vi "Auto_guider_queued.vi"() -> ()   [LabVIEW 2018]
uses:
  Global_Telescopio.vi
panel:
  out "respQ":refnum<queue>
  out "cmdQ":refnum<queue>
  in  "Case Constant\n(See Context Help) 2":bool
  in  "Case Constant\n(See Context Help)":bool=TRUE
  out "substring 3":string
  out "substring 2":string
  out "concatenated string":string
  out "substring":string
  out "result string":string
  in  "esc_placa":string="0.462"
  in  "guide_esp":string="S"
  in  "guide_cas":string="S"
  in  "guide_str":string="04/10/09  1:18:34\u000013 27 13\u0000-12 45 20\u0000"
  in  "guide_ang":string=" 281.52"
  in  "guide_nor":string="  11.53"
  in  "Tx_sts":u8[](array[numeric])=[22, 2, 1, 0, 83, 0, 0]
  out "rxsts 3":bool
  in  "SYN | ETX":u8[](array[numeric])=[22, 3] format="%02.0f"
  in  "tel_sts2":u8[](array[numeric])=[0, 0, 0] format="%02.0f"
  in  "Tx_ena":u8[](array[numeric])=[22, 2, 1, 0, 72, 0, 0] format="%02.0f"
  out "tel_sts1":bool[](array[boolean])=[TRUE, TRUE, TRUE, TRUE, FALSE, FALSE, TRUE]
  out "guide_dec":dbl format="%07.2g"
  out "guide_dir_ns":string
  out "guide_asc":dbl format="%07.2g"
  out "guide_dir_we":string
  in  "SYN | ACK":u8[](array[numeric])=[22, 6] format="%02.0f"
  out "rxsts":bool
  in  "Tx_nak":u8[](array[numeric])=[22, 21]
  out "Data rx guider":string
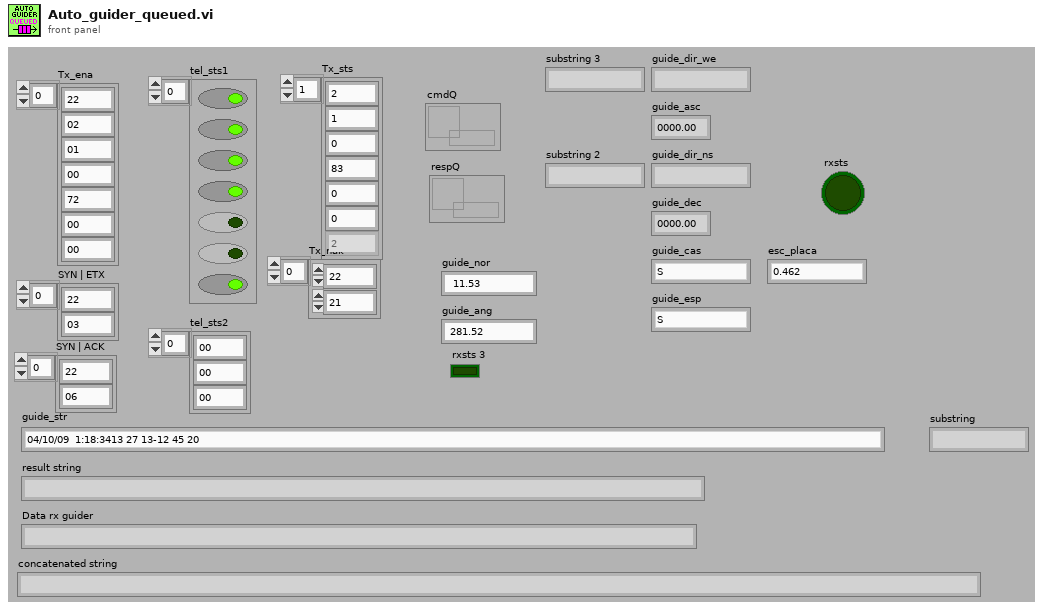
[diagram p1: front panel]
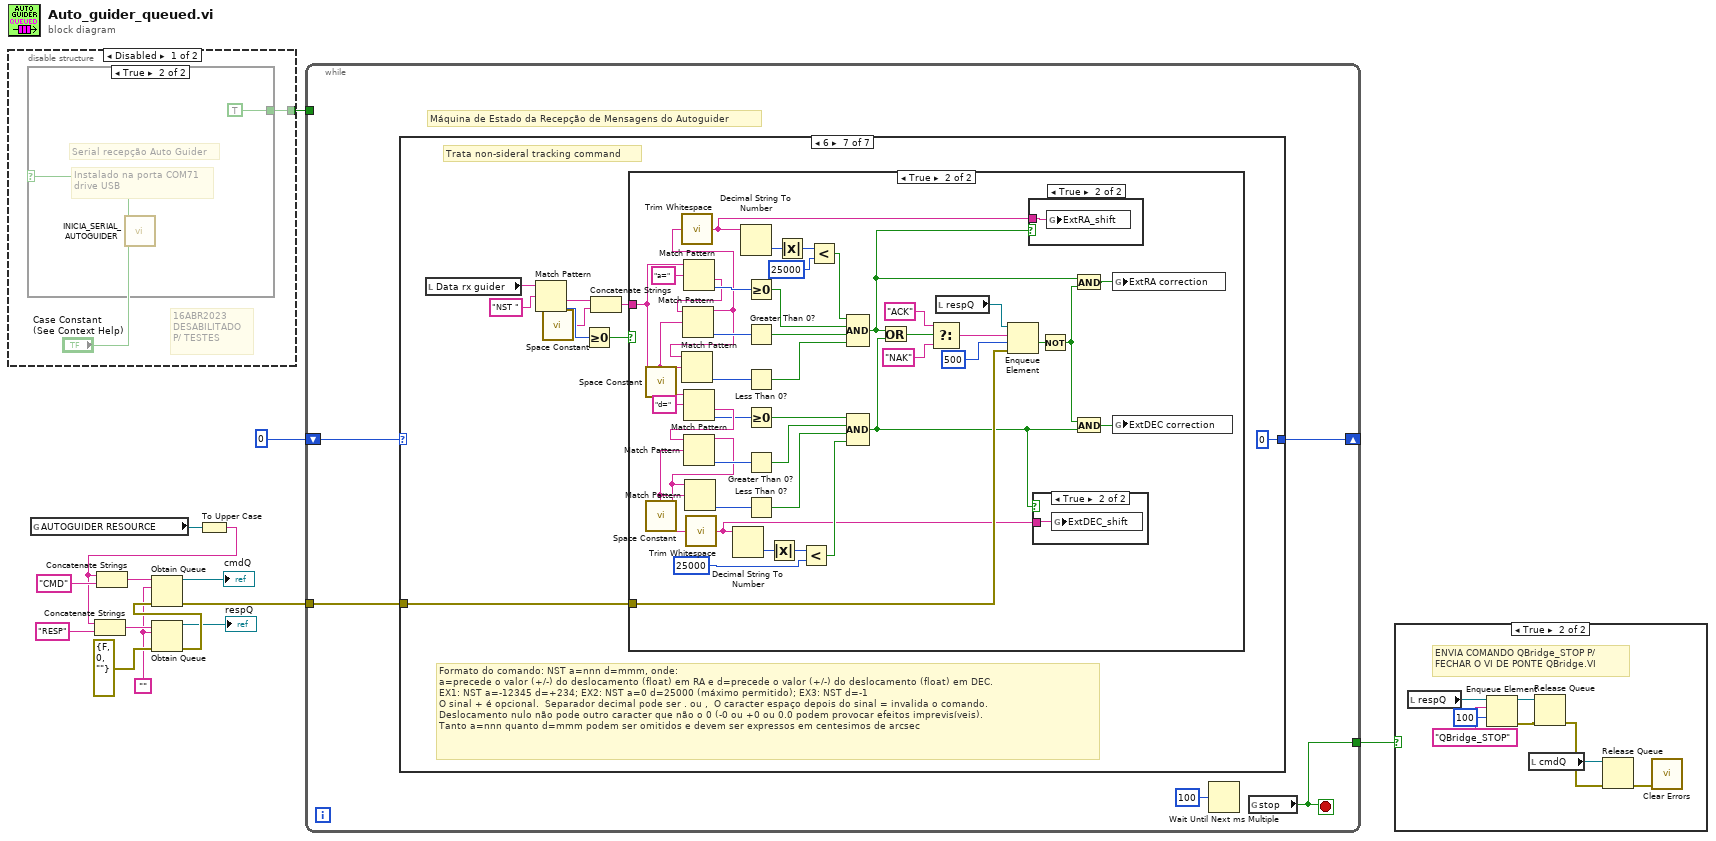
[diagram p0: block diagram]
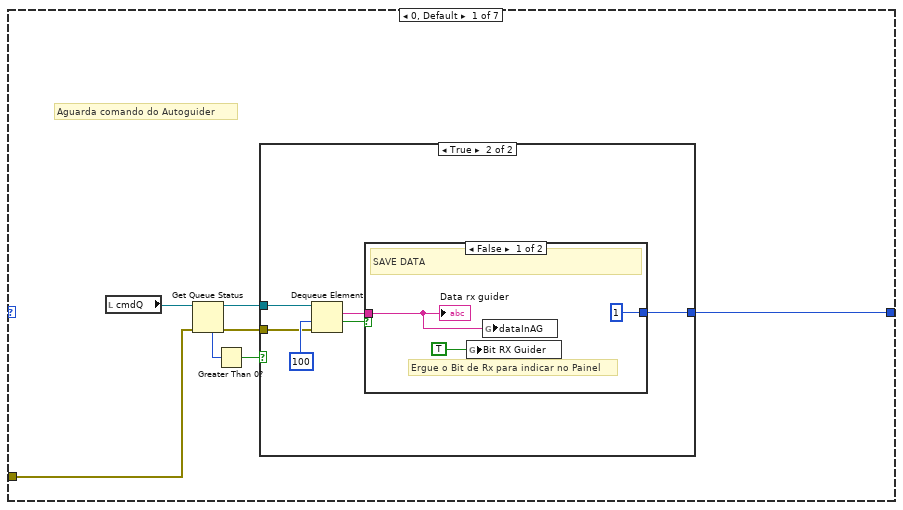
[diagram p5: hidden frame]
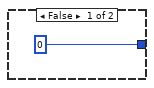
[diagram p6: hidden frame]
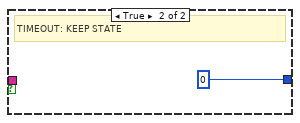
[diagram p7: hidden frame]
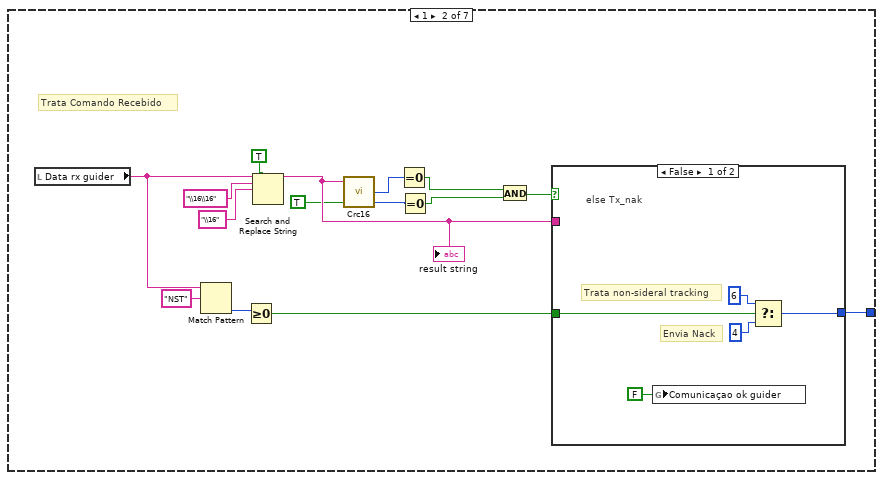
[diagram p8: hidden frame]
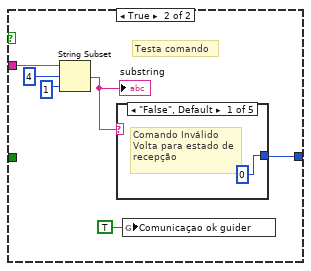
[diagram p9: hidden frame]
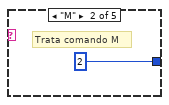
[diagram p10: hidden frame]
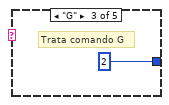
[diagram p11: hidden frame]
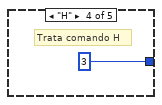
[diagram p12: hidden frame]
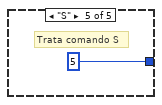
[diagram p13: hidden frame]
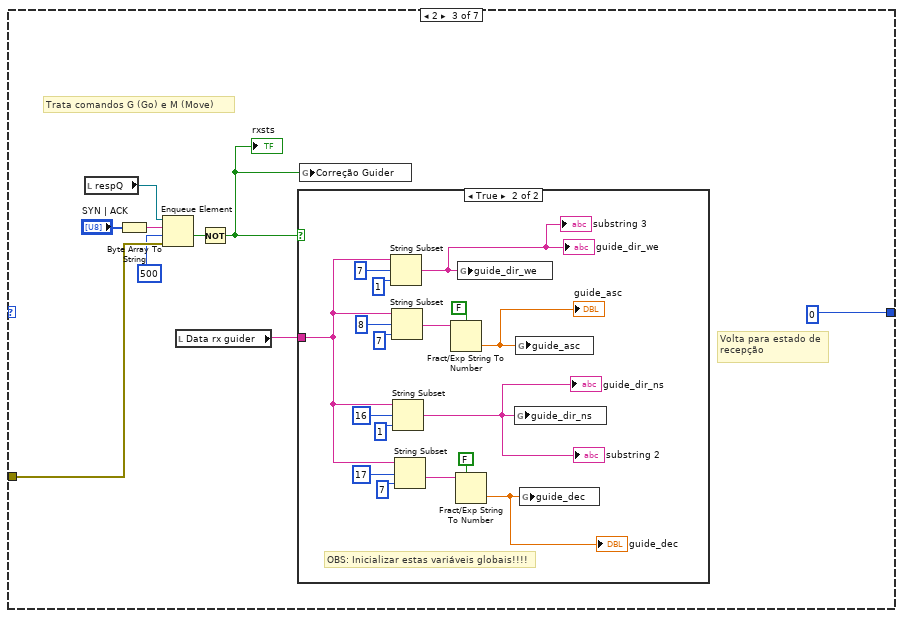
[diagram p14: hidden frame]
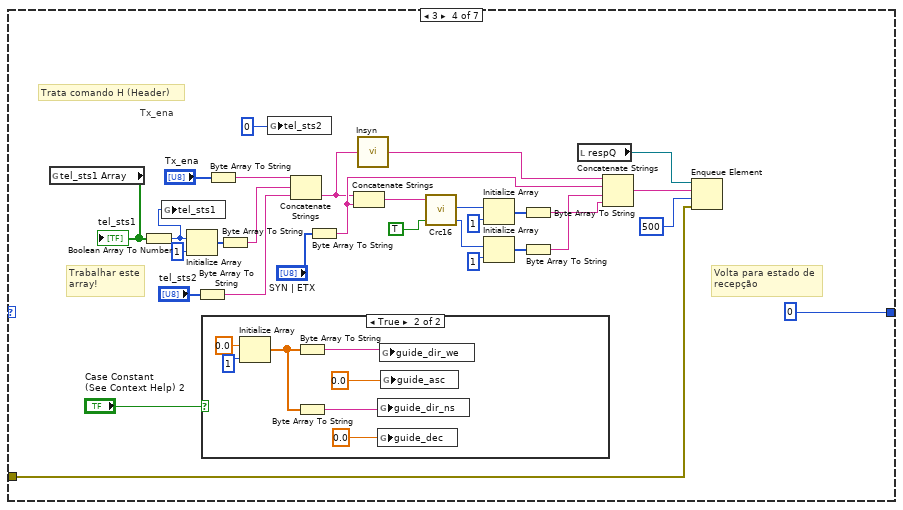
[diagram p16: hidden frame]
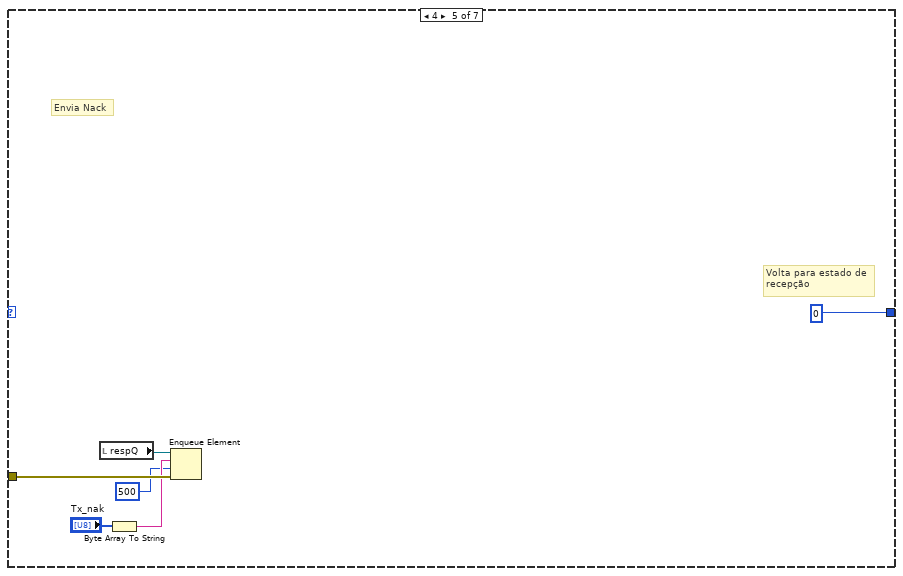
[diagram p18: hidden frame]
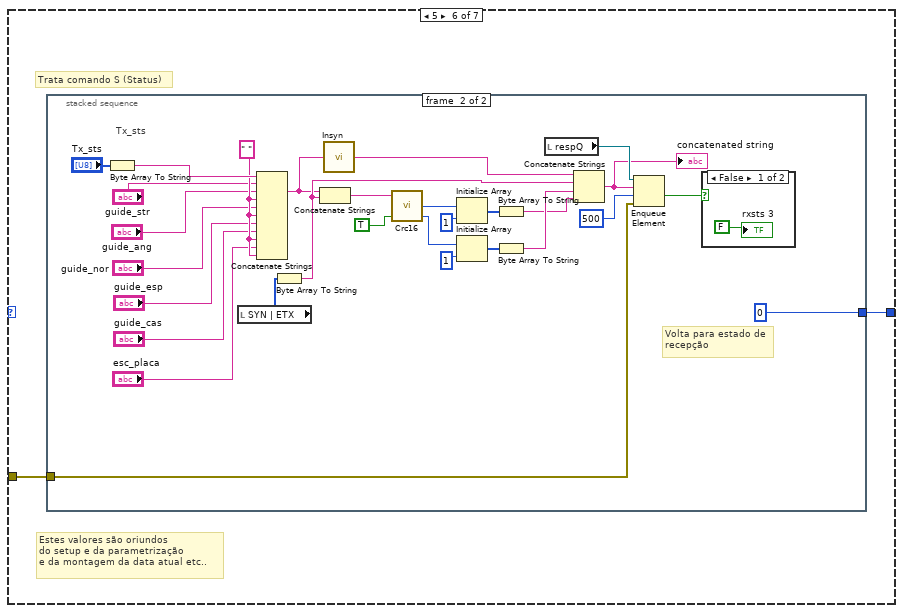
[diagram p19: hidden frame]
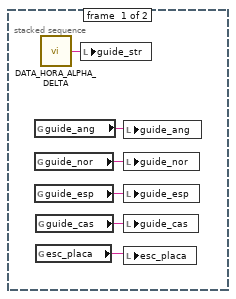
[diagram p20: hidden frame]
diagram:
  w2 = ""
  n1 = disable-structure shown="Disabled" {
    disable-tunnel: [w16 _] -> w14
    frame Disabled {
      # "16ABR2023\nDESABILITADO\nP/ TESTES"
      n2 = case shown="True" "Case Constant\n(See Context Help)" {
        tunnel: [_ TRUE] -> w16
        frame False {
        }
        frame True {
          # "Instalado na porta COM71\ndrive USB"
          # "Serial recepção Auto Guider"
          n3 = call "INICIA_SERIAL_AUTOGUIDER.vi"() -> ()  [unwired: 6 in, 1 out]
        }
      }
    }
    frame Enabled {
    }
  }
  n4 = global read "Global_Telescopio.vi" "AUTOGUIDER RESOURCE"() -> (w13:refnum<visa-resource-name>)
  n5 = To Upper Case(1:w13) -> (0:w10:string)
  n6 = Concatenate Strings(w10, "RESP" ("string")) -> (w9:string)
  n7 = Concatenate Strings(w10, "CMD" ("string")) -> (w8:string)
  n8 = Obtain Queue(name (unnamed)=w9, element data type=w2, error in (no error)=errorcluster {"status"=FALSE, "code"=0, "source"=""}) -> (queue out=→"respQ":refnum<queue>, error out=w6:errorcluster)  [unwired: 2 in, 1 out]
  n9 = Obtain Queue(name (unnamed)=w8, element data type=w2, error in (no error)=w6) -> (queue out=→"cmdQ":refnum<queue>, error out=w5:errorcluster)  [unwired: 2 in, 1 out]
  n10 = while {
    shift-right: [w21] -> _
    shift-left: 0 -> [w22]
    tunnel: w14 -> [_]
    tunnel: w5 -> [w20]
    tunnel: [w19] -> w1
    stop <- w19 stop-if-true
    # "Máquina de Estado da Recepção de Mensagens do Autoguider"
    n11 = case shown="6" w22 {
      tunnel: [w29 w56 0 0 0 w143 0] -> w21
      tunnel: w20 -> [w25 _ w77 w99 w138 w142 w180]
      frame 0, Default {
        # "Aguarda comando do Autoguider"
        n12 = local read "cmdQ"() -> (w24:refnum<queue>)
        n13 = Get Queue Status(queue=w24, error in (no error)=w25) -> (queue out=w28:refnum<queue>, error out=w27:errorcluster, # elements in queue=w26:i32)  [unwired: 1 in, 5 out]
        n14 = Greater Than 0?(x=w26) -> (x > 0?=w30:bool)
        n15 = case shown="True" w30 {
          tunnel: [0 w37] -> w29
          tunnel: w27 -> [_ w33]
          tunnel: w28 -> [_ w32]
          frame False {
          }
          frame True {
            n16 = Dequeue Element(queue=w32, timeout in ms (-1)=100, error in (no error)=w33) -> (element=w35:string, timed out?=w36:bool)  [unwired: 2 out]
            n17 = case shown="False" w36 {
              tunnel: [1 0] -> w37
              tunnel: w35 -> [w38 _]
              frame False {
                # "Ergue o Bit de Rx para indicar no Painel"
                # "SAVE DATA"
                n18 = global write "Global_Telescopio.vi" "Bit RX Guider"(TRUE) -> ()
                n19 = global write "Global_Telescopio.vi" "dataInAG"(w38) -> ()
                "Data rx guider" <- w38
              }
              frame True {
                # "TIMEOUT: KEEP STATE"
              }
            }
          }
        }
      }
      frame 1 {
        # "Trata Comando Recebido"
        n20 = local read "Data rx guider"() -> (w42:string)
        n21 = Match Pattern(string=w42, regular expression="NST") -> (offset past match=w44:i32)  [unwired: 1 in, 3 out]
        n22 = Greater Or Equal To 0?(x=w44) -> (x >= 0?=w43:bool)
        n23 = Search and Replace String(replace all?=TRUE ("replace all? (F)"), input string=w42, search string="\\16\\16", replace string="\\16" ("replace string (\"\")")) -> (result string=w52:string)  [unwired: 4 in, 3 out]
        "result string" <- w52
        n24 = call "Crc16.vi"("Habilita"=TRUE, "tx_rx_buf"=w52) -> ("crc_lo"=w49:u8, "crc_hi"=w50:u8)  [unwired: 1 in, 1 out]
        n25 = Equal To 0?(x=w50) -> (x = 0?=w46:bool)
        n26 = Equal To 0?(x=w49) -> (x = 0?=w47:bool)
        n27 = And(x=w46, y=w47) -> (x .and. y?=w48:bool)
        n28 = case shown="False" w48 {
          tunnel: [w57 w67] -> w56
          tunnel: w52 -> [_ w66]
          tunnel: w43 -> [w60 _]
          frame False {
            # "Trata non-sideral tracking"
            # "else Tx_nak"
            # "Envia Nack"
            n29 = global write "Global_Telescopio.vi" "Comunicaçao ok guider"(FALSE ("Comunicaçao ok guider")) -> ()
            n30 = Select(t=6, s=w60, f=4) -> (s? t:f=w57:i32)
          }
          frame True {
            # "Testa comando"
            n31 = String Subset(string=w66, offset (0)=4, length (rest)=1 ("length (rest)")) -> (substring=w63:string)
            "substring" <- w63
            n32 = case shown="\"False\", Default" w63 {
              tunnel: [0 2 2 3 5] -> w67
              frame "False", Default {
                # "Comando Inválido\nVolta para estado de\nrecepção"
              }
              frame "M" {
                # "Trata comando M"
              }
              frame "G" {
                # "Trata comando G"
              }
              frame "H" {
                # "Trata comando H"
              }
              frame "S" {
                # "Trata comando S"
              }
            }
            n33 = global write "Global_Telescopio.vi" "Comunicaçao ok guider"(TRUE ("Comunicaçao ok guider")) -> ()
          }
        }
      }
      frame 2 {
        # "Volta para estado de\nrecepção"
        # "Trata comandos G (Go) e M (Move)"
        n34 = local read "respQ"() -> (w78:refnum<queue>)
        n35 = Byte Array To String(unsigned byte array="SYN | ACK") -> (string=w79:string)
        n36 = Enqueue Element(queue=w78, element=w79, timeout in ms (-1)=500, error in (no error)=w77) -> (timed out?=w75:bool)  [unwired: 2 out]
        n37 = local read "Data rx guider"() -> (w80:string)
        n38 = Not(x=w75) -> (.not. x?=w74:bool)
        "rxsts" <- w74
        n39 = case shown="True" w74 {
          tunnel: w80 -> [_ w94]
          frame False {
          }
          frame True {
            # "OBS: Inicializar estas variáveis globais!!!!"
            n40 = String Subset(string=w94, offset (0)=7, length (rest)=1 ("length (rest)")) -> (substring=w85:string)
            "guide_dir_we" <- w85
            "substring 3" <- w85
            n41 = String Subset(string=w94, offset (0)=8, length (rest)=7 ("length (rest)")) -> (substring=w89:string)
            n42 = String Subset(string=w94, offset (0)=16, length (rest)=1 ("length (rest)")) -> (substring=w83:string)
            "guide_dir_ns" <- w83
            "substring 2" <- w83
            n43 = String Subset(string=w94, offset (0)=17, length (rest)=7 ("length (rest)")) -> (substring=w88:string)
            n44 = Fract/Exp String To Number(use system decimal point (T)=FALSE, string=w89) -> (number=w84:dbl)  [unwired: 2 in, 1 out]
            "guide_asc" <- w84
            n45 = Fract/Exp String To Number(use system decimal point (T)=FALSE, string=w88) -> (number=w82:dbl)  [unwired: 2 in, 1 out]
            "guide_dec" <- w82
            n46 = global write "Global_Telescopio.vi" "guide_dir_we"(w85) -> ()
            n47 = global write "Global_Telescopio.vi" "guide_dir_ns"(w83) -> ()
            n48 = global write "Global_Telescopio.vi" "guide_asc"(w84) -> ()
            n49 = global write "Global_Telescopio.vi" "guide_dec"(w82) -> ()
          }
        }
        n50 = global write "Global_Telescopio.vi" "Correção Guider"(w74) -> ()
      }
      frame 3 {
        # "Volta para estado de\nrecepção"
        # "Trabalhar este\narray!"
        # "Tx_ena"
        # "Trata comando H (Header)"
        n51 = global read "Global_Telescopio.vi" "tel_sts1 Array"() -> (w105:bool[])
        "tel_sts1" <- w105
        n52 = Boolean Array To Number(Boolean array=w105) -> (number=w106:u32)
        n53 = global write "Global_Telescopio.vi" "tel_sts1"(w106) -> ()
        n54 = Initialize Array(w106, 1 ("dimension size")) -> (w113:u32[])
        n55 = Byte Array To String(unsigned byte array="tel_sts2") -> (string=w126:string)
        n56 = case shown="True" "Case Constant\n(See Context Help) 2" {
          frame False {
          }
          frame True {
            n57 = Initialize Array(0.0 ("element"), 1 ("dimension size")) -> (w133:dbl[])
            n58 = Byte Array To String(unsigned byte array=w133) -> (string=w132:string)
            n59 = Byte Array To String(unsigned byte array=w133) -> (string=w130:string)
            n60 = global write "Global_Telescopio.vi" "guide_dir_ns"(w130) -> ()
            n61 = global write "Global_Telescopio.vi" "guide_dec"(0.0 ("guide_dec")) -> ()
            n62 = global write "Global_Telescopio.vi" "guide_dir_we"(w132) -> ()
            n63 = global write "Global_Telescopio.vi" "guide_asc"(0.0 ("guide_asc")) -> ()
          }
        }
        n64 = Byte Array To String(unsigned byte array="Tx_ena") -> (string=w124:string)
        n65 = Byte Array To String(unsigned byte array=w113) -> (string=w114:string)
        n66 = global write "Global_Telescopio.vi" "tel_sts2"(0) -> ()
        n67 = Concatenate Strings(w124, w114, w126) -> (w110:string)
        n68 = Byte Array To String(unsigned byte array="SYN | ETX") -> (string=w128:string)
        n69 = Concatenate Strings(w110, w128) -> (w109:string)
        n70 = call "Insyn.vi"("txbuf"=w110) -> ("txbuf OUT"=w111:string)
        n71 = call "Crc16.vi"("Habilita"=TRUE, "tx_rx_buf"=w109) -> ("crc_lo"=w118:u8, "crc_hi"=w116:u8)  [unwired: 1 in, 1 out]
        n72 = Initialize Array(w116, 1 ("dimension size")) -> (w120:u8[])
        n73 = Initialize Array(w118, 1 ("dimension size")) -> (w119:u8[])
        n74 = Byte Array To String(unsigned byte array=w120) -> (string=w121:string)
        n75 = Byte Array To String(unsigned byte array=w119) -> (string=w122:string)
        n76 = local read "respQ"() -> (w102:refnum<queue>)
        n77 = Concatenate Strings(w111, w128, w122, w121) -> (w101:string)
        n78 = Enqueue Element(queue=w102, element=w101, timeout in ms (-1)=500, error in (no error)=w99) -> ()  [unwired: 3 out]
      }
      frame 4 {
        # "Volta para estado de\nrecepção"
        # "Envia Nack"
        n79 = local read "respQ"() -> (w139:refnum<queue>)
        n80 = Byte Array To String(unsigned byte array="Tx_nak") -> (string=w137:string)
        n81 = Enqueue Element(queue=w139, element=w137, timeout in ms (-1)=500, error in (no error)=w138) -> ()  [unwired: 3 out]
      }
      frame 5 {
        # "Estes valores são oriundos\ndo setup e da parametrização\ne da montagem da data atual etc.."
        # "Trata comando S (Status)"
        n82 = stacked-sequence {
          tunnel: [_ 0] -> w143
          tunnel: w142 -> [_ w153]
          frame #0 {
            n83 = global read "Global_Telescopio.vi" "guide_ang"() -> (w148:string)
            n84 = global read "Global_Telescopio.vi" "guide_nor"() -> (w147:string)
            n85 = global read "Global_Telescopio.vi" "guide_esp"() -> (w146:string)
            n86 = global read "Global_Telescopio.vi" "guide_cas"() -> (w145:string)
            n87 = global read "Global_Telescopio.vi" "esc_placa"() -> (w144:string)
            n88 = call "DATA_HORA_ALPHA_DELTA.vi"() -> ("SAIDA"=w149:string)  [unwired: 2 in]
            n89 = local write "guide_str"(w149) -> ()
            n90 = local write "guide_ang"(w148) -> ()
            n91 = local write "guide_nor"(w147) -> ()
            n92 = local write "guide_esp"(w146) -> ()
            n93 = local write "guide_cas"(w145) -> ()
            n94 = local write "esc_placa"(w144) -> ()
          }
          frame #1 {
            w167 = " " ("string")
            # "Volta para estado de\nrecepção"
            # "Tx_sts"
            n95 = Byte Array To String(unsigned byte array="Tx_sts") -> (string=w178:string)
            n96 = local read "SYN | ETX"() -> (w157:u8[])
            n97 = Concatenate Strings(w178, "guide_str", "guide_ang", w167, "guide_nor", w167, "guide_esp", "guide_cas", w167, "esc_placa", w167) -> (w165:string)
            n98 = Byte Array To String(unsigned byte array=w157) -> (string=w176:string)
            n99 = Concatenate Strings(w165, w176) -> (w164:string)
            n100 = call "Insyn.vi"("txbuf"=w165) -> ("txbuf OUT"=w166:string)
            n101 = call "Crc16.vi"("Habilita"=TRUE, "tx_rx_buf"=w164) -> ("crc_lo"=w172:u8, "crc_hi"=w173:u8)  [unwired: 1 in, 1 out]
            n102 = Initialize Array(w173, 1 ("dimension size")) -> (w171:u8[])
            n103 = Initialize Array(w172, 1 ("dimension size")) -> (w170:u8[])
            n104 = Byte Array To String(unsigned byte array=w171) -> (string=w174:string)
            n105 = Byte Array To String(unsigned byte array=w170) -> (string=w175:string)
            n106 = local read "respQ"() -> (w155:refnum<queue>)
            n107 = Concatenate Strings(w166, w176, w175, w174) -> (w154:string)
            "concatenated string" <- w154
            n108 = Enqueue Element(queue=w155, element=w154, timeout in ms (-1)=500, error in (no error)=w153) -> (timed out?=w150:bool)  [unwired: 2 out]
            n109 = case shown="False" w150 {
              frame False {
                "rxsts 3" <- FALSE ("rxsts")
              }
              frame True {
              }
            }
          }
        }
      }
      frame 6 {
        # "Formato do comando: NST a=nnn d=mmm, onde:\na=precede o valor (+/-) do deslocamento (float) em RA e d=precede o valor (+/-) do deslocamento (float) em DEC.\nEX1: NST a=-12345 d=+234; EX2: NST a=0 d=25000 (máximo permitido); EX3: NST d=-1\nO sinal + é opcional.  Separador decimal pode ser . ou ,  O caracter espaço depois do sinal = invalida o comando. \nDeslocamento nulo não pode outro caracter que não o 0 (-0 ou +0 ou 0.0 podem provocar efeitos imprevisíveis).\nTanto a=nnn quanto d=mmm podem ser omitidos e devem ser expressos em centesimos de arcsec"
        # "Trata non-sideral tracking command"
        n110 = local read "Data rx guider"() -> (w188:string)
        n111 = Match Pattern(string=w188, regular expression="NST ") -> (after substring=w184:string, offset past match=w186:i32)  [unwired: 1 in, 2 out]
        n112 = call <vilib>:"Space Constant.vi"() -> ("String"=w183:string)
        n113 = Greater Or Equal To 0?(x=w186) -> (x >= 0?=w185:bool)
        n114 = Concatenate Strings(w184, w183) -> (w182:string)
        n115 = case shown="True" w185 {
          tunnel: w182 -> [_ w223]
          tunnel: w180 -> [_ w216]
          frame False {
          }
          frame True {
            n116 = call <vilib>:"Space Constant.vi"() -> ("String"=w211:string)
            n117 = call <vilib>:"Space Constant.vi"() -> ("String"=w206:string)
            n118 = Match Pattern(string=w223, regular expression="a=") -> (after substring=w229:string, offset past match=w232:i32)  [unwired: 1 in, 2 out]
            n119 = Match Pattern(string=w229, regular expression=w211) -> (before substring=w212:string, offset past match=w230:i32)  [unwired: 1 in, 2 out]
            n120 = call <vilib>:"Trim Whitespace.vi"("string"=w212) -> ("trimmed string"=w192:string)  [unwired: 1 in]
            n121 = Match Pattern(string=w212, regular expression=w211) -> (offset past match=w210:i32)  [unwired: 1 in, 3 out]
            n122 = Match Pattern(string=w223, regular expression="d=") -> (after substring=w226:string, offset past match=w224:i32)  [unwired: 1 in, 2 out]
            n123 = Match Pattern(string=w226, regular expression=w206) -> (before substring=w202:string, offset past match=w225:i32)  [unwired: 1 in, 2 out]
            n124 = Match Pattern(string=w202, regular expression=w206) -> (offset past match=w205:i32)  [unwired: 1 in, 3 out]
            n125 = call <vilib>:"Trim Whitespace.vi"("string"=w202) -> ("trimmed string"=w190:string)  [unwired: 1 in]
            n126 = Decimal String To Number(string=w190) -> (number=w203:i32)  [unwired: 2 in, 1 out]
            n127 = Decimal String To Number(string=w192) -> (number=w197:i32)  [unwired: 2 in, 1 out]
            n128 = Greater Or Equal To 0?(x=w232) -> (x >= 0?=w227:bool)
            n129 = Greater Than 0?(x=w230) -> (x > 0?=w228:bool)
            n130 = Less Than 0?(x=w210) -> (x < 0?=w209:bool)
            n131 = Greater Or Equal To 0?(x=w224) -> (x >= 0?=w208:bool)
            n132 = Greater Than 0?(x=w225) -> (x > 0?=w207:bool)
            n133 = Less Than 0?(x=w205) -> (x < 0?=w204:bool)
            n134 = Absolute Value(x=w203) -> (abs(x)=w201:i32)
            n135 = Absolute Value(x=w197) -> (abs(x)=w198:i32)
            n136 = Less?(x=w201, y=25000 ("abs(x)")) -> (x < y?=w199:bool)
            n137 = Less?(x=w198, y=25000 ("abs(x)")) -> (x < y?=w195:bool)
            n138 = Compound Arithmetic op=AND(w195, w227, w228, w209) -> (w191:bool)
            n139 = Compound Arithmetic op=AND(w208, w207, w204, w199) -> (w189:bool)
            n140 = Or(x=w191, y=w189) -> (x .or. y?=w219:bool)
            n141 = Select(t="ACK", s=w219, f="NAK") -> (s? t:f=w194:string)
            n142 = local read "respQ"() -> (w221:refnum<queue>)
            n143 = Enqueue Element(queue=w221, element=w194, timeout in ms (-1)=500, error in (no error)=w216) -> (timed out?=w215:bool)  [unwired: 2 out]
            n144 = case shown="True" w191 {
              tunnel: w192 -> [_ w234]
              frame False {
              }
              frame True {
                n145 = global write "Global_Telescopio.vi" "ExtRA_shift"(w234) -> ()
              }
            }
            n146 = case shown="True" w189 {
              tunnel: w190 -> [_ w233]
              frame False {
              }
              frame True {
                n147 = global write "Global_Telescopio.vi" "ExtDEC_shift"(w233) -> ()
              }
            }
            n148 = Not(x=w215) -> (.not. x?=w193:bool)
            n149 = And(x=w191, y=w193) -> (x .and. y?=w214:bool)
            n150 = And(x=w193, y=w189) -> (x .and. y?=w213:bool)
            n151 = global write "Global_Telescopio.vi" "ExtRA correction"(w214) -> ()
            n152 = global write "Global_Telescopio.vi" "ExtDEC correction"(w213) -> ()
          }
        }
      }
    }
    n153 = Wait Until Next ms Multiple(millisecond multiple=u32 100) -> ()  [unwired: 1 out]
    n154 = global read "Global_Telescopio.vi" "stop"() -> (w19:bool)
  }
  n155 = case shown="True" w1 {
    frame False {
    }
    frame True {
      # "ENVIA COMANDO QBridge_STOP P/\nFECHAR O VI DE PONTE QBridge.VI"
      n156 = local read "respQ"() -> (w242:refnum<queue>)
      n157 = Enqueue Element(queue=w242, element="QBridge_STOP" ("x"), timeout in ms (-1)=100) -> (queue out=w240:refnum<queue>, error out=w238:errorcluster)  [unwired: 1 in, 1 out]
      n158 = local read "cmdQ"() -> (w241:refnum<queue>)
      n159 = Release Queue(queue=w240, error in (no error)=w238) -> (error out=w237:errorcluster)  [unwired: 1 in, 2 out]
      n160 = Release Queue(queue=w241, error in (no error)=w237) -> (error out=w236:errorcluster)  [unwired: 1 in, 2 out]
      n161 = call <vilib>:"Clear Errors.vi"("error in (no error)"=w236) -> ()  [unwired: 5 in, 2 out]
    }
  }
